vi "calc_delta.vi"(1 "C":dbl=2.0, 2 "B":dbl=3.0, 3 "A":dbl=1.0) -> (0 "Delta":dbl=1.0)   [LabVIEW 2022 SP3]
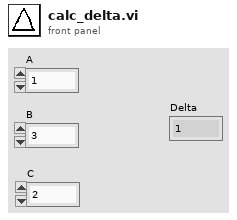
[diagram p1: front panel]
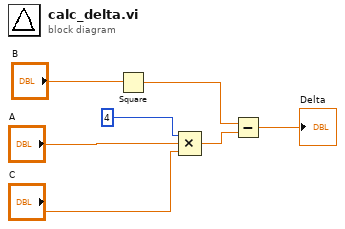
[diagram p0: block diagram]
diagram:
  n1 = Square(x="B") -> (x^2=w6:dbl)
  n2 = Compound Arithmetic op=MULTIPLY(i8 4 ("y"), "A", "C") -> (w3:dbl)
  n3 = Subtract(x=w6, y=w3) -> (x-y=→"Delta":dbl)
